vi "csmdoc_import_all_csm_VI_description_doc.vi"(11 "Path":path=path "D:/github/JKI-State-Machine-Plus/.doc/VI Description.md") -> ()   [LabVIEW 2017, in "csmdoc.lvlib"]
uses:
  csmdoc.lvlib
panel:
  in  "Error in":errorcluster caption="Error in (no error)"
  out "error out":errorcluster
  out "Array":path[](array[path])
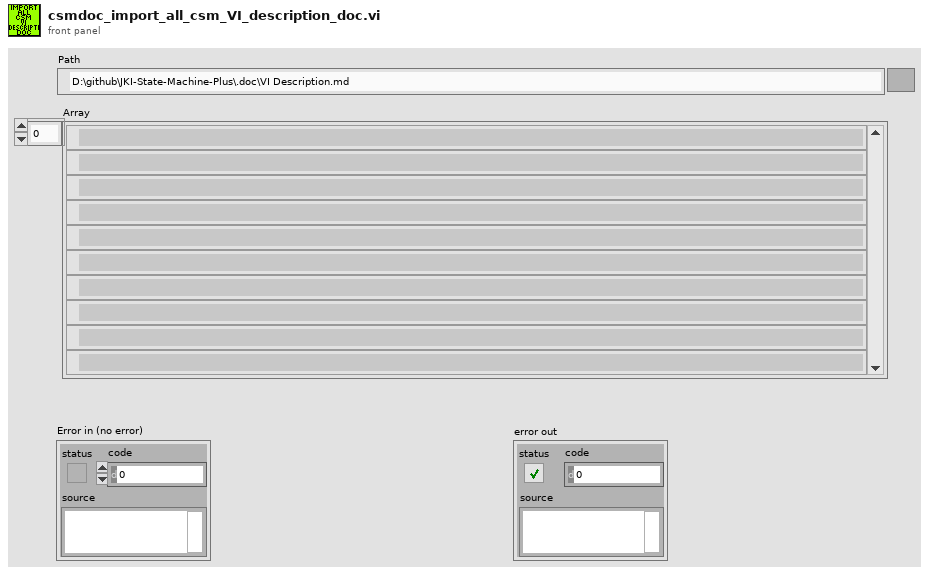
[diagram p1: front panel]
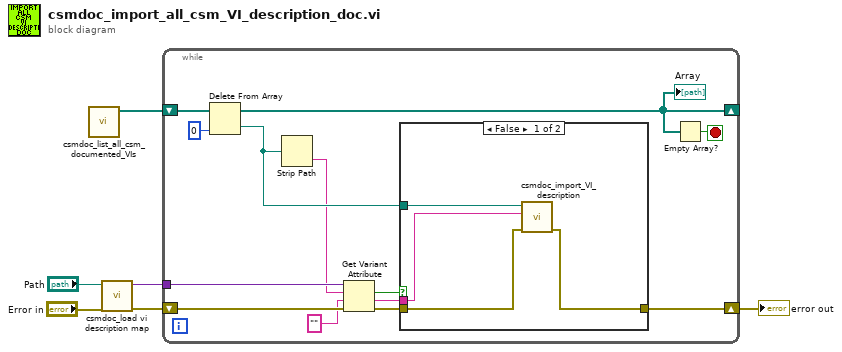
[diagram p0: block diagram]
diagram:
  n1 = call "csmdoc_list_all_csm_documented_VIs.vi"() -> ("Array"=w6:path[])  [unwired: 11 in]
  n2 = call "csmdoc_load vi description map.vi"("Error in"="Error in", "Path"="Path") -> ("Error out"=w3:errorcluster, "variant"=w5:variant)  [unwired: 7 in, 1 out]
  n3 = while {
    shift-right: [w16] -> _
    shift-left: w6 -> [w18]
    tunnel: w5 -> [w14]
    shift-right: [w9] -> w2
    shift-left: w3 -> [w11]
    stop <- w17 stop-if-true
    n4 = Delete From Array(array=w18, index=0) -> (deleted portion=w19:path, array with subset deleted=w16:path[])  [unwired: 1 in]
    "Array" <- w16
    n5 = Strip Path(path=w19) -> (name=w13:string)  [unwired: 1 out]
    n6 = Get Variant Attribute(Variant=w14, name=w13, default value (empty Variant)="" ("String"), error in=w11) -> (found=w12:bool, value=w7:string, error out=w10:errorcluster)  [unwired: 1 out]
    n7 = case shown="False" w12 {
      tunnel: w19 -> [w23 _]
      tunnel: w10 -> [w22 w24]
      tunnel: [w21 w24] -> w9
      tunnel: w7 -> [w20 _]
      frame False {
        n8 = call "csmdoc_import_VI_description.vi"("error in (no error)"=w22, "string"=w20, "Path"=w23) -> ("error out"=w21:errorcluster)  [unwired: 8 in]
      }
      frame True {
      }
    }
    n9 = Empty Array?(array=w16) -> (empty?=w17:bool)
  }
  "error out" <- w2
